vi "Array Average 2x2 array.vi"(4 "Array to Average":dbl[][](array[numeric])) -> (0 "min value":dbl, 1 "Average":dbl, 2 "max value":dbl)   [LabVIEW 2016]
panel:
  out "size":i32
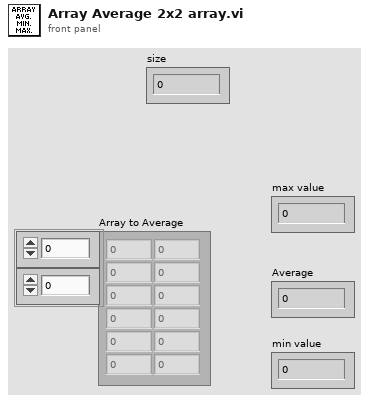
[diagram p1: front panel]
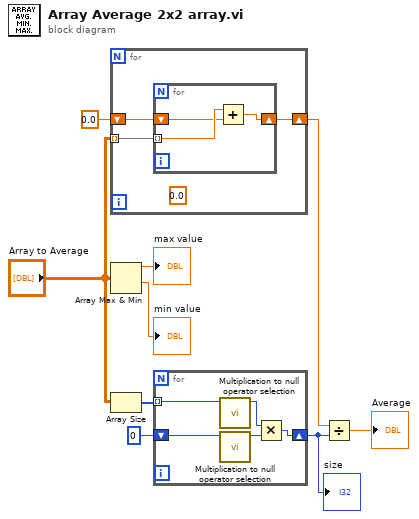
[diagram p0: block diagram]
diagram:
  n1 = for {
    tunnel: "Array to Average" -> [w12] mode=indexing
    shift-right: [w10] -> w3
    shift-left: 0.0 -> [w11]
    (unwired) 0.0
    n2 = for {
      tunnel: w12 -> [w15] mode=indexing
      shift-right: [w14] -> w10
      shift-left: w11 -> [w13]
      n3 = Add(x=w15, y=w13) -> (x+y=w14:dbl)
    }
  }
  n4 = Array Max & Min(array="Array to Average") -> (max value=→"max value":dbl, min value=→"min value":dbl)  [unwired: 2 out]
  n5 = Array Size(array="Array to Average") -> (size(s)=w7:i32[])
  n6 = for {
    tunnel: w7 -> [w18] mode=indexing
    shift-right: [w20] -> w2
    shift-left: 0 -> [w19]
    n7 = call "Multiplication to null operator selection.vi"("Numeric Control"=w18) -> ("t"=w17:i32)  [unwired: 10 in]
    n8 = call "Multiplication to null operator selection.vi"("Numeric Control"=w19) -> ("t"=w16:i32)  [unwired: 10 in]
    n9 = Multiply(x=w17, y=w16) -> (x*y=w20:i32)
  }
  "size" <- w2
  n10 = Divide(x=w3, y=w2) -> (x/y=→"Average":dbl)
